vi "CALC_LIM_SEGM_TYPE.vi"(0 "VISA IN":refnum<visa-resource-name>, 1 "Segment number":i32, 2 "Segment Limit":string(combo)="OFF", 5 "error in":errorcluster, 7 "Channel":i32) -> (14 "VISA Out":refnum<visa-resource-name>, 19 "error out":errorcluster)   [LabVIEW 2018, in "PNA-X.lvlib"]
doc: "CALCulate<cnum>:LIMit:SEGMent<snum>:TYPE <char> \n1524\n\n(Read-Write) Sets the type of limit segment. \nSee Critical Note \nParameters \n<cnum> Channel number of the measurement. There must be a selected measurement \non that channel. If unspecified, <cnum> is set to 1. \n<snum> Segment number. Choose any number between: \n1 and 100 \nIf unspecified, value is set to 1. \n<char> Choose from: \nLMAX - a MAX limit segment. Any response data exceeding the MAX value \nwill fail. \nLMIN - a MIN limit segment. Any response data below the MIN value will \nfail. \nOFF - the limit segment (display and testing) is turned OFF. \nExamples CALC:LIM:SEGM:TYPE LMIN \ncalculate2:limit:segment3:type lmax \nQuery Syntax CALCulate<cnum>:LIMit:SEGMent<snum>:TYPE? \nReturn Type Character \nDefault OFF"
uses:
  PNA-X.lvlib
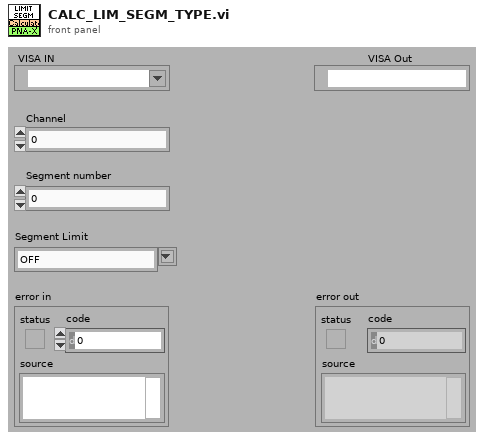
[diagram p1: front panel]
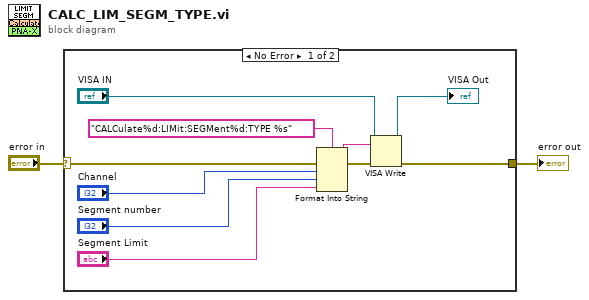
[diagram p0: block diagram]
diagram:
  n1 = case shown="No Error" "error in" {
    selector: "error in" -> [w12 w13]
    tunnel: [w7 w13] -> w1
    frame No Error {
      n2 = Format Into String(format string="CALCulate%d:LIMit:SEGMent%d:TYPE %s" ("Cmdline"), error in=w12, "Channel", "Segment number", "Segment Limit") -> (resulting string=w10:string, error out=w11:errorcluster)  [unwired: 1 in]
      n3 = VISA Write(VISA resource name="VISA IN", write buffer=w10, error in (no error)=w11) -> (VISA resource name out=→"VISA Out":refnum<visa-resource-name>, error out=w7:errorcluster)  [unwired: 1 out]
    }
    frame Error {
    }
  }
  "error out" <- w1
